vi "add dynamic member to class by name.vi"(8 "error in":errorcluster, 9 "name":string, 10 "LVClassLibrary in":refnum<vi>, 11 "Application in":refnum<vi>) -> (0 "error out":errorcluster)   [LabVIEW 2013, in "NISE Tools Scripting.lvlib"]
uses:
  NISE Tools Scripting.lvlib
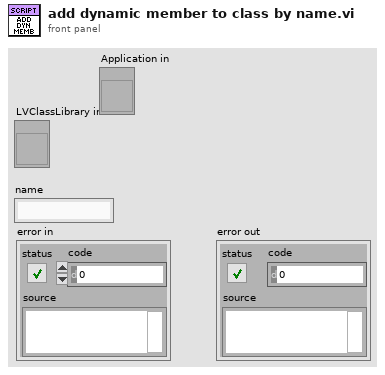
[diagram p1: front panel]
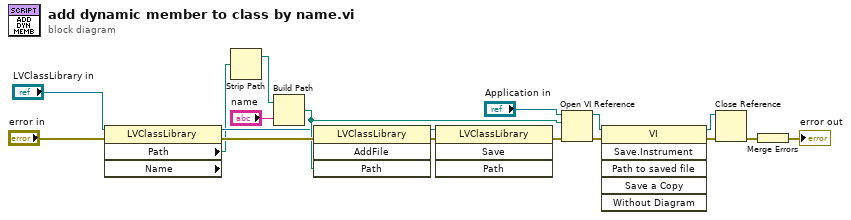
[diagram p0: block diagram]
diagram:
  n1 = property class="LVClassLibrary" props=["Path", "Name"](reference="LVClassLibrary in", error in="error in") -> (reference out=w7:refnum<vi>, error out=w10:errorcluster, "Path"=w3:path)  [unwired: 1 out]
  n2 = Strip Path(path=w3) -> (stripped path=w9:path)  [unwired: 1 out]
  n3 = Build Path(base path=w9, name or relative path="name") -> (appended path=w8:path)
  n4 = invoke class="LVClassLibrary" method="AddFile"(reference=w7, error in=w10, "Path"=w8) -> (reference out=w12:refnum<vi>, error out=w11:errorcluster)  [unwired: 1 in, 2 out]
  n5 = invoke class="LVClassLibrary" method="Save"(reference=w12, error in=w11) -> (error out=w5:errorcluster)  [unwired: 2 in, 3 out]
  n6 = Open VI Reference(application reference (local)="Application in", vi path=w8, error in (no error)=w5) -> (vi reference=w1:refnum<vi>, error out=w2:errorcluster)  [unwired: 3 in]
  n7 = invoke class="VI" method="Save.Instrument"(reference=w1, error in=w2) -> (reference out=w17:refnum<vi>, error out=w16:errorcluster)  [unwired: 4 in, 4 out]
  n8 = Close Reference(reference=w17, error in (no error)=w16) -> (error out=w15:errorcluster)
  n9 = Merge Errors(w15) -> (→"error out":errorcluster)
